vi "Channel and Position.vi"(11 "Menu event":refnum<user-event>) -> ()   [LabVIEW 2009]
panel:
  in  "Select Channel":u32(slide)
  in  "Volts/Div":u32(knob)
  in  "Time Base":u32(knob)
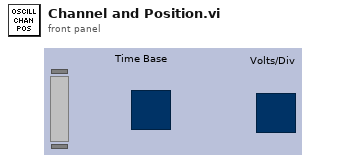
[diagram p1: front panel]
types:
  T1 = enum16{"All Elements", "Channel", "Source", "Level", "Slope", "Time Base", "Volts / Div"}
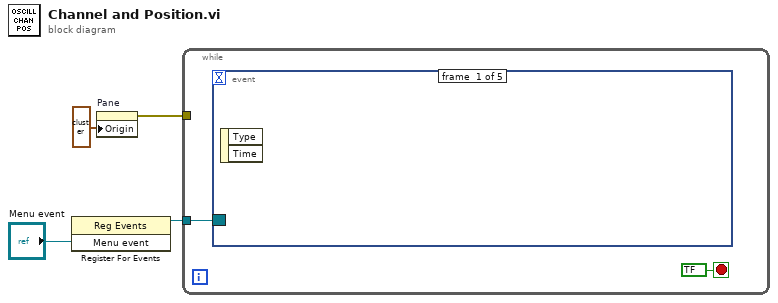
[diagram p0: block diagram]
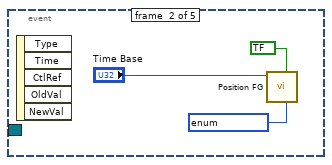
[diagram p2: hidden frame]
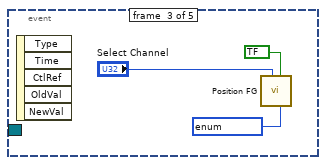
[diagram p3: hidden frame]
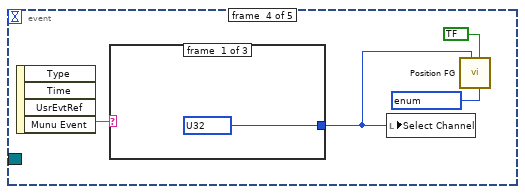
[diagram p4: hidden frame]
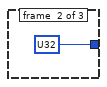
[diagram p5: hidden frame]
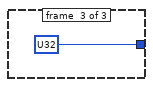
[diagram p6: hidden frame]
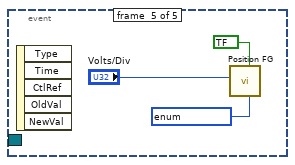
[diagram p7: hidden frame]
diagram:
  n1 = register-events("Menu event") -> (reference out=w3:refnum<event-registration>)  [unwired: 2 in, 1 out]
  n2 = property on="Pane" class="Pane"("Origin"=cluster{"Horizontal":i16, "Vertical":i16} ?) -> (error out=w1:errorcluster)  [unwired: 2 in, 1 out]
  n3 = while {
    tunnel: w3 -> [w5]
    tunnel: w1 -> [_]
    stop <- bool ? stop-if-true
    n4 = event shown="[3] <Menu event>: User Event" {
      selector: w5 -> [_ _ _ _ _]
      dyn-events: _ -> [_ _ _ _ _]
      timeout: _ -> [_ _ _ _ _]
      event #0 {
        n5 = event-data() -> ()  [unwired: 1 in, 2 out]
      }
      event #1 {
        n6 = event-data() -> ()  [unwired: 1 in, 5 out]
        n7 = call "Position FG.vi"("Parameter"=T1 ?, "Get / Set (T=Set)"=bool ?, "Time Base In"="Time Base") -> ()  [unwired: 8 in, 1 out]
      }
      event #2 {
        n8 = event-data() -> ()  [unwired: 1 in, 5 out]
        n9 = call "Position FG.vi"("Parameter"=T1 ?, "Get / Set (T=Set)"=bool ?, "Channel In"="Select Channel") -> ()  [unwired: 8 in, 1 out]
      }
      event #3 {
        n10 = event-data() -> ("Munu Event"=w16:string)  [unwired: 1 in, 3 out]
        n11 = case shown="\"Channel A\"" w16 {
          tunnel: [w17 w18 w19] -> w13
          frame #0 {
            w17 = u32 ? items=["A & B", "B", "A"] ("Select Channel")
          }
          frame #1 {
            w18 = u32 ? items=["A & B", "B", "A"] ("Select Channel")
          }
          frame #2 {
            w19 = u32 ? items=["A & B", "B", "A"] ("Select Channel")
          }
        }
        n12 = local write "Select Channel"(w13) -> ()
        n13 = call "Position FG.vi"("Parameter"=T1 ?, "Get / Set (T=Set)"=bool ?, "Channel In"=w13) -> ()  [unwired: 8 in, 1 out]
      }
      event #4 {
        n14 = event-data() -> ()  [unwired: 1 in, 5 out]
        n15 = call "Position FG.vi"("Parameter"=T1 ?, "Get / Set (T=Set)"=bool ?, "Volts / Div In"="Volts/Div") -> ()  [unwired: 8 in, 1 out]
      }
    }
  }
